vi "Machs2-11-15.vi"(0 "Heizen?Mach1":bool, 1 "Heizen?Mach2":bool, 2 "PIDMach1":T1 {"proportional gain (Kc)" format="%.11g"; "integral gain (Kc*Ts/Ti)" format="%.11g"; "derivative gain (Kc*Td/Ts)" format="%.11g"}, 3 "PIDMach2":T1 {"proportional gain (Kc)" format="%.11g"; "integral gain (Kc*Ts/Ti)" format="%.11g"; "derivative gain (Kc*Td/Ts)" format="%.11g"}, 4 "Umax[V]Mach1":fxp<+/-,16,4> format="%.14g", 5 "Umax[V]Mach2":fxp<+/-,16,4> format="%.14g", 6 "USetp[V]Mach1":fxp<+/-,16,4> format="%.14g", 7 "USetp[V]Mach2":fxp<+/-,16,4> format="%.14g", 10 "Per[us]Mach":u16 caption="Periode Mach [us]", 12 "vor der Messung [us]Mach":u16=200, 14 "wie viele Messwerte?Mach":u16, 16 "Abstand zwischen Messungen [us]Mach":u16 caption="Abstand zwischen Messungen Mach [us]") -> (20 "U[V]Mach1":fxp<+/-,16,4> format="%.25g", 22 "U[V]Mach2":fxp<+/-,16,4> format="%.25g")   [LabVIEW 2010]
uses:
  <vilib>/eio/EIONode/EIONode.xnode
  <vilib>/rvi/eio/nirviEIOImplementation/nirviEIOImplementation.xnode
  <vilib>/rvi/eio/common/nirviEmuClasses.ctl
  <vilib>/rvi/FXPMathLib/FxpAdd/XNode/nifxpmath_Add.xnode
  <vilib>/rvi/FXPMathLib/FxpAdd/subVIs/nifxpmath_Add_SimConfig.ctl
  <vilib>/fxp/LVFixedPointQuantizationPolicyTypeDef.ctl
  <vilib>/fxp/LVFixedPointOverflowPolicyTypeDef.ctl
  <vilib>/rvi/FXPMathLib/FxpDiv/XNode/nifxpmath_Div.xnode
  <vilib>/rvi/FXPMathLib/FxpDiv/subVIs/nifxpmath_Div_SimConfig.ctl
  <vilib>/rvi/FXPMathLib/FxpMul/XNode/nifxpmath_Multiplier.xnode
  <vilib>/rvi/FXPMathLib/FxpMul/subVIs/nifxpmath_Mul_SimConfig.ctl
  <vilib>/rvi/FXPMathLib/FxpSqrt/XNode/nifxpmath_Sqrt.xnode
  <vilib>/rvi/FXPMathLib/FxpSqrt/subVIs/nifxpmath_Sqrt_SimConfig.ctl
  <vilib>/rvi/FXPMathLib/FxpConvert/XNode/nifxpmath_Convert.xnode
  <vilib>/rvi/FXPMathLib/FxpConvert/subVIs/nifxpmath_Convert_SimConfig.ctl
  <vilib>/addons/control/pid/fpga.llb/XNode/niFpgaPID.xnode
  <vilib>/rvi/eio/common/nirviEmuTemplateMethod_noerrors.vi
  <vilib>/rvi/FXPMathLib/FxpAdd/simVIs/DllFxpAddTemp_sub.vi
  <vilib>/rvi/FXPMathLib/FxpDiv/simVIs/DllFxpDivTemp_sub.vi
  <vilib>/rvi/FXPMathLib/FxpMul/simVIs/DllFxpMulTemp_sub.vi
  <vilib>/rvi/FXPMathLib/FxpSqrt/simVIs/DllSqrtTemp_sub.vi
  <vilib>/rvi/FXPMathLib/FxpConvert/simVIs/DllFxpConvertTemp_sub.vi
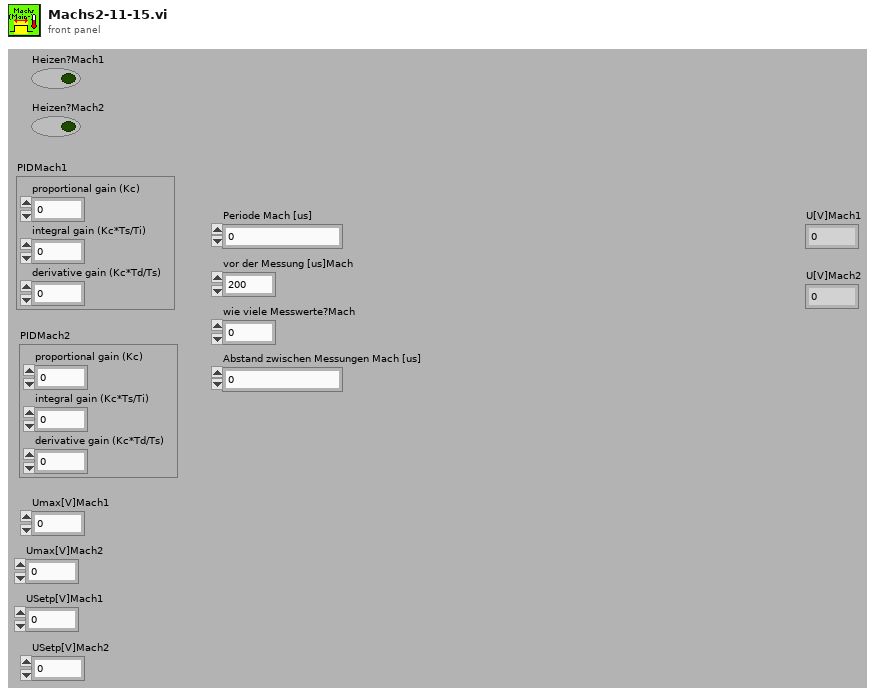
[diagram p1: front panel]
types:
  T1 = cluster{"proportional gain (Kc)":fxp<+/-,16,8>, "integral gain (Kc*Ts/Ti)":fxp<+/-,16,8>, "derivative gain (Kc*Td/Ts)":fxp<+/-,16,8>}
  T2 = cluster{"output high":fxp<+/-,16,4>, "output low":fxp<+/-,16,4>}
  T3 = typedef "nirviEmuClasses.ctl" = enum16{"IO Read", "IO Write", "Method", "Property Read", "Property Write"}
  T4 = cluster{"proportional gain (Kc)":i16, "integral gain (Kc*Ts/Ti)":i16, "derivative gain (Kc*Td/Ts)":i16}
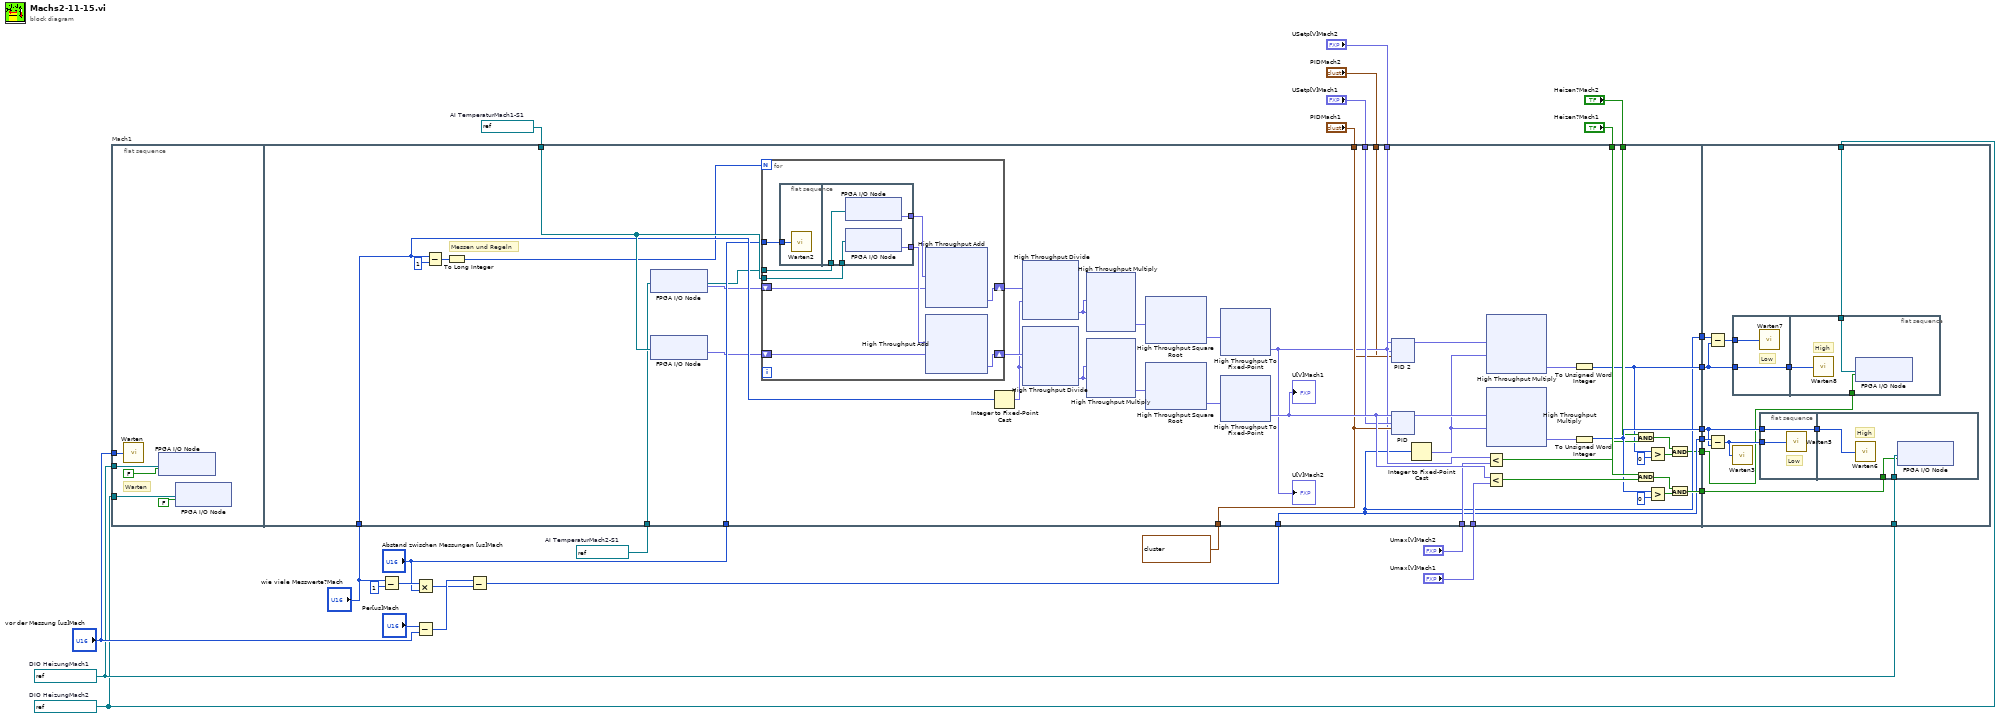
[diagram p0: block diagram]
diagram:
  w1 = refnum<k21> "Mod6/DIO17"  # DIO HeizungMach2
  w11 = refnum<k21> "Mod1/AI7"  # AI TemperaturMach2-S1
  w25 = refnum<k21> "Mod1/AI5"  # AI TemperaturMach1-S1
  w2 = refnum<k21> "Mod6/DIO28"  # DIO HeizungMach1
  n1 = flat-sequence "Mach1" {
    tunnel: "vor der Messung [us]Mach" -> [w33]
    tunnel: w2 -> [w32]
    tunnel: w1 -> [w29]
    tunnel: w25 -> [w102]
    tunnel: "Abstand zwischen Messungen [us]Mach" -> [w99]
    tunnel: "wie viele Messwerte?Mach" -> [w100]
    tunnel: [w80] -> w28
    tunnel: [w90] -> w27
    tunnel: [w57] -> w26
    tunnel: w14 -> [w57]
    tunnel: "Umax[V]Mach1" -> [w85]
    tunnel: "USetp[V]Mach1" -> [w84]
    tunnel: "Heizen?Mach1" -> [w83]
    tunnel: "PIDMach1" -> [w82]
    tunnel: w11 -> [w70]
    tunnel: "USetp[V]Mach2" -> [w63]
    tunnel: T2 {"output high"=1.0, "output low"=0.0} ("output range") -> [w62]
    tunnel: "PIDMach2" -> [w61]
    tunnel: "Umax[V]Mach2" -> [w60]
    tunnel: "Heizen?Mach2" -> [w59]
    tunnel: [w58] -> w5
    tunnel: [w57] -> w4
    tunnel: [w56] -> w3
    tunnel: w28 -> [w597]
    tunnel: w27 -> [w594]
    tunnel: w26 -> [w599]
    tunnel: w5 -> [w591]
    tunnel: w4 -> [w592]
    tunnel: w3 -> [w589]
    tunnel: w2 -> [w595]
    tunnel: w1 -> [w588]
    frame #0 {
      # "Warten"
      n2 = call "Warten"("Count(uSec)"=w33) -> ()  [unwired: 1 out]
      n3 = xnode "FPGA I/O Node"("I/O Item"=FALSE, "FPGA I/O In"=w32) -> ()  [unwired: 1 out]
      n4 = xnode "FPGA I/O Node"("I/O Item"=FALSE, "FPGA I/O In"=w29) -> ()  [unwired: 1 out]
    }
    frame #1 {
      # "Messen und Regeln"
      n5 = Subtract(x=w100, y=u16 1) -> (x-y=w98:u16)
      n6 = To Long Integer(number=w98) -> (32bit integer=w97:i32)
      n7 = xnode "FPGA I/O Node"("FPGA I/O In"=w70) -> ("I/O Item"=w69:fxp<+/-,26,5>, "FPGA I/O Out"=w68:refnum<k21>)
      n8 = xnode "FPGA I/O Node"("FPGA I/O In"=w102) -> ("I/O Item"=w81:fxp<+/-,26,5>)  [unwired: 1 out]
      n9 = for {
        N: w97 -> [_]
        shift-right: [w434] -> w101
        shift-left: w81 -> [w435]
        tunnel: w99 -> [w438]
        tunnel: w102 -> [w437]
        shift-right: [w431] -> w67
        shift-left: w69 -> [w432]
        tunnel: w68 -> [w433]
        n10 = flat-sequence {
          tunnel: w438 -> [w499]
          tunnel: w437 -> [w503]
          tunnel: [w502] -> w436
          tunnel: w433 -> [w501]
          tunnel: [w500] -> w430
          frame #0 {
            n11 = call "Warten2"("Count(uSec)"=w499) -> ()  [unwired: 1 out]
          }
          frame #1 {
            n12 = xnode "FPGA I/O Node"("FPGA I/O In"=w501) -> ("I/O Item"=w500:fxp<+/-,26,5>)  [unwired: 1 out]
            n13 = xnode "FPGA I/O Node"("FPGA I/O In"=w503) -> ("I/O Item"=w502:fxp<+/-,26,5>)  [unwired: 1 out]
          }
        }
        n14 = xnode "High Throughput Add"("x"=w430, "y"=w432) -> ("x+y"=w431:fxp<+/-,32,11>)
        n15 = xnode "High Throughput Add"("x"=w436, "y"=w435) -> ("x+y"=w434:fxp<+/-,32,11>)
      }
      n16 = Integer to Fixed-Point Cast ("Integer in Festkomma umwandeln")(integer=w100) -> (fixed-point=w66:fxp<+/-,8,8>)  [unwired: 1 in]
      n17 = xnode "High Throughput Divide"("x"=w67, "y"=w66) -> ("x/y"=w73:fxp<+/-,16,4>)
      n18 = xnode "High Throughput Divide"("x"=w101, "y"=w66) -> ("x/y"=w89:fxp<+/-,16,4>)
      n19 = xnode "High Throughput Multiply"("x"=w73, "y"=w73) -> ("x*y"=w72:fxp<+,32,8>)
      n20 = xnode "High Throughput Multiply"("x"=w89, "y"=w89) -> ("x*y"=w88:fxp<+,32,8>)
      n21 = xnode "High Throughput Square Root"("x"=w72) -> ("sqrt(x)"=w71:fxp<+,16,4>)
      n22 = xnode "High Throughput Square Root"("x"=w88) -> ("sqrt(x)"=w87:fxp<+,16,4>)
      n23 = xnode "High Throughput To Fixed-Point"("x"=w71) -> ("y"=w64:fxp<+/-,16,4>)
      "U[V]Mach2" <- w64
      n24 = xnode "High Throughput To Fixed-Point"("x"=w87) -> ("y"=w86:fxp<+/-,16,4>)
      "U[V]Mach1" <- w86
      n25 = xnode ("PID 2")("process variable"=w64, "setpoint"=w63, "PID gains"=w61, "output range"=w62) -> ("output"=w79:fxp<+/-,16,4>)  [unwired: 1 in]
      n26 = xnode ("PID")("process variable"=w86, "setpoint"=w84, "PID gains"=w82, "output range"=w62) -> ("output"=w96:fxp<+/-,16,4>)  [unwired: 1 in]
      n27 = Integer to Fixed-Point Cast ("Integer in Festkomma umwandeln")(integer=w57) -> (fixed-point=w65:fxp<+,16,16>)  [unwired: 1 in]
      n28 = Less?(x=w64, y=w60) -> (x < y?=w77:bool)
      n29 = Less?(x=w86, y=w85) -> (x < y?=w94:bool)
      n30 = xnode "High Throughput Multiply"("x"=w79, "y"=w65) -> ("x*y"=w78:fxp<+/-,16,16>)
      n31 = xnode "High Throughput Multiply"("x"=w96, "y"=w65) -> ("x*y"=w95:fxp<+/-,16,16>)
      n32 = To Unsigned Word Integer(number=w78) -> (unsigned 16bit integer=w58:u16)
      n33 = To Unsigned Word Integer(number=w95) -> (unsigned 16bit integer=w80:u16)
      n34 = And(x=w59, y=w77) -> (x .and. y?=w75:bool)
      n35 = And(x=w83, y=w94) -> (x .and. y?=w92:bool)
      n36 = Greater?(x=w58, y=u16 0) -> (0:w74:bool)
      n37 = Greater?(x=w80, y=u16 0) -> (0:w91:bool)
      n38 = And(x=w75, y=w74) -> (x .and. y?=w56:bool)
      n39 = And(x=w92, y=w91) -> (x .and. y?=w90:bool)
    }
    frame #2 {
      n40 = Subtract(x=w592, y=w591) -> (x-y=w590:u16)
      n41 = Subtract(x=w599, y=w597) -> (x-y=w598:u16)
      n42 = flat-sequence {
        tunnel: w590 -> [w601]
        tunnel: w591 -> [w600]
        tunnel: [w600] -> w593
        tunnel: w593 -> [w604]
        tunnel: w588 -> [w603]
        tunnel: w589 -> [w602]
        frame #0 {
          # "Low"
          n43 = call "Warten7"("Count(uSec)"=w601) -> ()  [unwired: 1 out]
        }
        frame #1 {
          # "High"
          n44 = call "Warten8"("Count(uSec)"=w604) -> ()  [unwired: 1 out]
          n45 = xnode "FPGA I/O Node"("I/O Item"=w602, "FPGA I/O In"=w603) -> ()  [unwired: 1 out]
        }
      }
      n46 = call "Warten3"("Count(uSec)"=w598) -> ()  [unwired: 1 out]
      n47 = flat-sequence {
        tunnel: w598 -> [w617]
        tunnel: w597 -> [w616]
        tunnel: [w616] -> w596
        tunnel: w596 -> [w620]
        tunnel: w595 -> [w619]
        tunnel: w594 -> [w618]
        frame #0 {
          # "Low"
          n48 = call "Warten5"("Count(uSec)"=w617) -> ()  [unwired: 1 out]
        }
        frame #1 {
          # "High"
          n49 = call "Warten6"("Count(uSec)"=w620) -> ()  [unwired: 1 out]
          n50 = xnode "FPGA I/O Node"("I/O Item"=w618, "FPGA I/O In"=w619) -> ()  [unwired: 1 out]
        }
      }
    }
  }
  n51 = Subtract(x="wie viele Messwerte?Mach", y=u16 1) -> (x-y=w23:u16)
  n52 = Multiply(x=w23, y="Abstand zwischen Messungen [us]Mach") -> (x*y=w21:u16)
  n53 = Subtract(x="Per[us]Mach", y="vor der Messung [us]Mach") -> (x-y=w22:u16)
  n54 = Subtract(x=w22, y=w21) -> (x-y=w14:u16)
